vi "Autonomous Independent.vi"() -> ()   [LabVIEW 2018]
doc: "This VI is called when autonomous begins, and will automatically be terminated when autonomous ends. You can carry out timed or sensor driven robot movement independently without needing to return to the caller."
uses:
  <vilib>/Rock Robotics/SystemInterfaces/spilib/spi_bus.ctl
  <vilib>/Rock Robotics/WPI/Utilities/WPI_GetSetVariantRefNum.vi
  <vilib>/Rock Robotics/Network Tables/NT Read String.vi
  <vilib>/Rock Robotics/Network Tables/NT Write Numeric Array.vi
  <vilib>/Rock Robotics/WPI/RobotDrive/WPI_RobotDriveArcadeDrive_Standard(NoSaturation).vi
  <vilib>/Rock Robotics/WPI/Gyro/WPI_GyroXRS450_SPI_Open.vi
panel:
  out "Degrees 2":dbl(knob) scale=0.0..360.0
  in  "Angle 2":dbl=1000.0 min=50.0 max=20000.0 format="%#_13g"
  in  "Angle 1":dbl=1000.0 min=50.0 max=20000.0 format="%#_13g"
  out "Device Found":bool
  in  "SPI Bus":T1
  in  "Sample Rate (Hz)":dbl=1000.0 min=50.0 max=20000.0 format="%#_13g"
  out "Degrees":dbl(knob) scale=0.0..360.0
  in  "Reset Angle?":bool
  out "Calibrated?":bool
  # "This shows wiring for the Analog Devices XRS450 gyro.  It can be plugged directly into the SPI port."
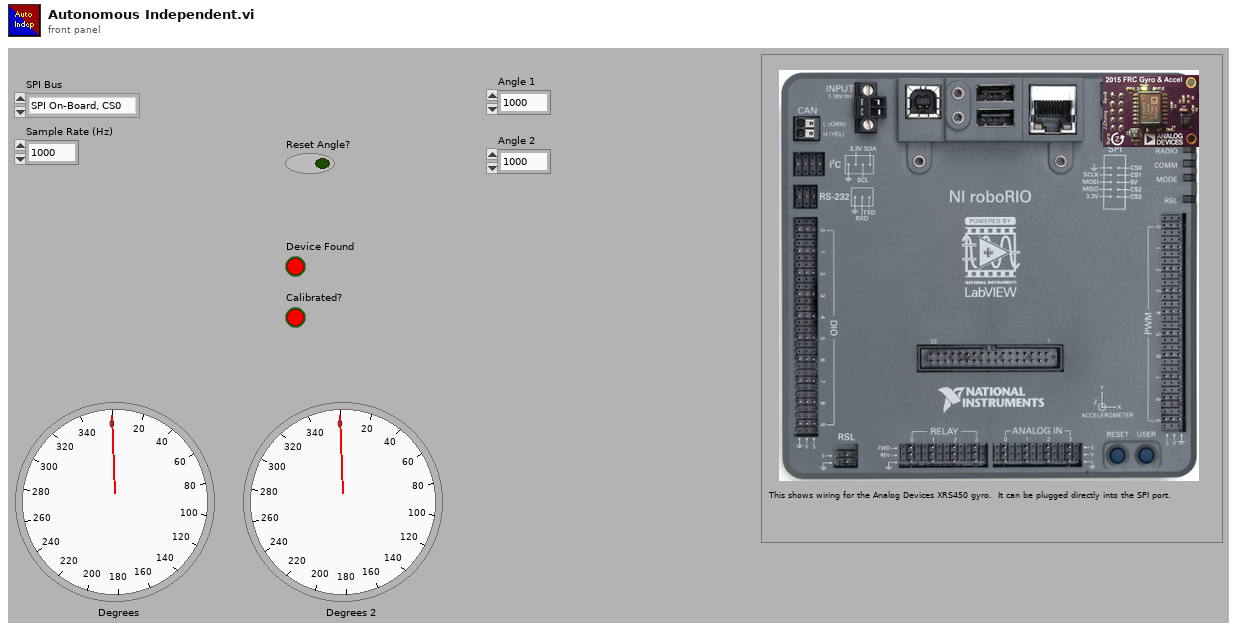
[diagram p1: front panel]
types:
  T1 = typedef "spi_bus.ctl" = enum16{"SPI On-Board, CS0", "SPI On-Board, CS1", "SPI On-Board, CS2", "SPI On-Board, CS3", "SPI MXP", "Invalid"}
  T2 = typedef "WPI_JoystickDevRef.ctl" = cluster{"Device":T3}
  T3 = typedef "WPI_JoystickDeviceEnum.ctl" = enum16{"USB 0", "USB 1", "USB 2", "USB 3", "USB 4", "USB 5"}
  T4 = typedef "WPI_RobotDriveDevRef.ctl" = cluster{"DevStatus":errorcluster, "Motors[]":T5[], "Square Inputs":bool, "Max Output":dbl}
  T5 = typedef "WPI_MotorControlDeviceRef.ctl" = cluster{"DeviceStatus":errorcluster, "Type":T6, "PWM":cluster{"PWM Channel":T7, "DeadBand":T8}, "CAN":cluster{"Device Number":u8, "SetOutput VI Ref":variant, "GetOutput VI Ref":variant, "Enable VI Ref":variant, "Disable VI Ref":variant, "Data":variant}, "Invert":bool, "DIO PWM":cluster{"PWM \"Enable\" Channel":T7, "DIOChannel":T9, "PWM Rate":dbl}}
  T6 = typedef "WPI_MotorControlType.ctl" = enum16{"PWM", "CAN", "DIO PWM"}
  T7 = typedef "FPGA_DIOPWMChannel.ctl" = enum8{"PWM 0", "PWM 1", "PWM 2", "PWM 3", "PWM 4", "PWM 5", "PWM 6", "PWM 7", "PWM 8", "PWM 9", "PWM MXP 0", "PWM MXP 1", "PWM MXP 2", "PWM MXP 3", "PWM MXP 4", "PWM MXP 5", "PWM MXP 6", "PWM MXP 7", "PWM MXP 8", "PWM MXP 9", "Invalid"}
  T8 = typedef "WPI_PWMDeadband.ctl" = cluster{"Name":string, "maxPositivePwm":i32, "minPositivePwm":i32, "centerPwm":i32, "maxNegativePwm":i32, "minNegativePwm":i32, "angularRange":u16}
  T9 = typedef "FPGA_DIOChannel.ctl" = enum8{"DIO 0", "DIO 1", "DIO 2", "DIO 3", "DIO 4", "DIO 5", "DIO 6", "DIO 7", "DIO 8", "DIO 9", "DIO MXP 0", "DIO MXP 1", "DIO MXP 2", "DIO MXP 3", "DIO MXP 4", "DIO MXP 5", "DIO MXP 6", "DIO MXP 7", "DIO MXP 8", "DIO MXP 9", "DIO MXP 10", "DIO MXP 11", "DIO MXP 12", "DIO MXP 13", "DIO MXP 14", "DIO MXP 15", "SPI Port CS1", "SPI Port CS2", "SPI Port CS3", "SPI Port MISO", "SPI Port MOSI", "Invalid"}
  T10 = typedef "WPI_GyroDevRef.ctl" = cluster{"DevStatus":errorcluster, "Analog Channel":T11, "Gain (VoltsPerDegree/Second)":dbl, "Gyro Type":enum16{"Analog", "XRS450"}, "Handle":i32, "SPI Bus":T1, "Device Found":bool, "Sample Rate":dbl, "Calibrate On Open":bool, "Offset":dbl}
  T11 = typedef "FPGA_AIChannel.ctl" = enum8{"AI 0", "AI 1", "AI 2", "AI 3", "AI MXP 0", "AI MXP 1", "AI MXP 2", "AI MXP 3", "Invalid"}
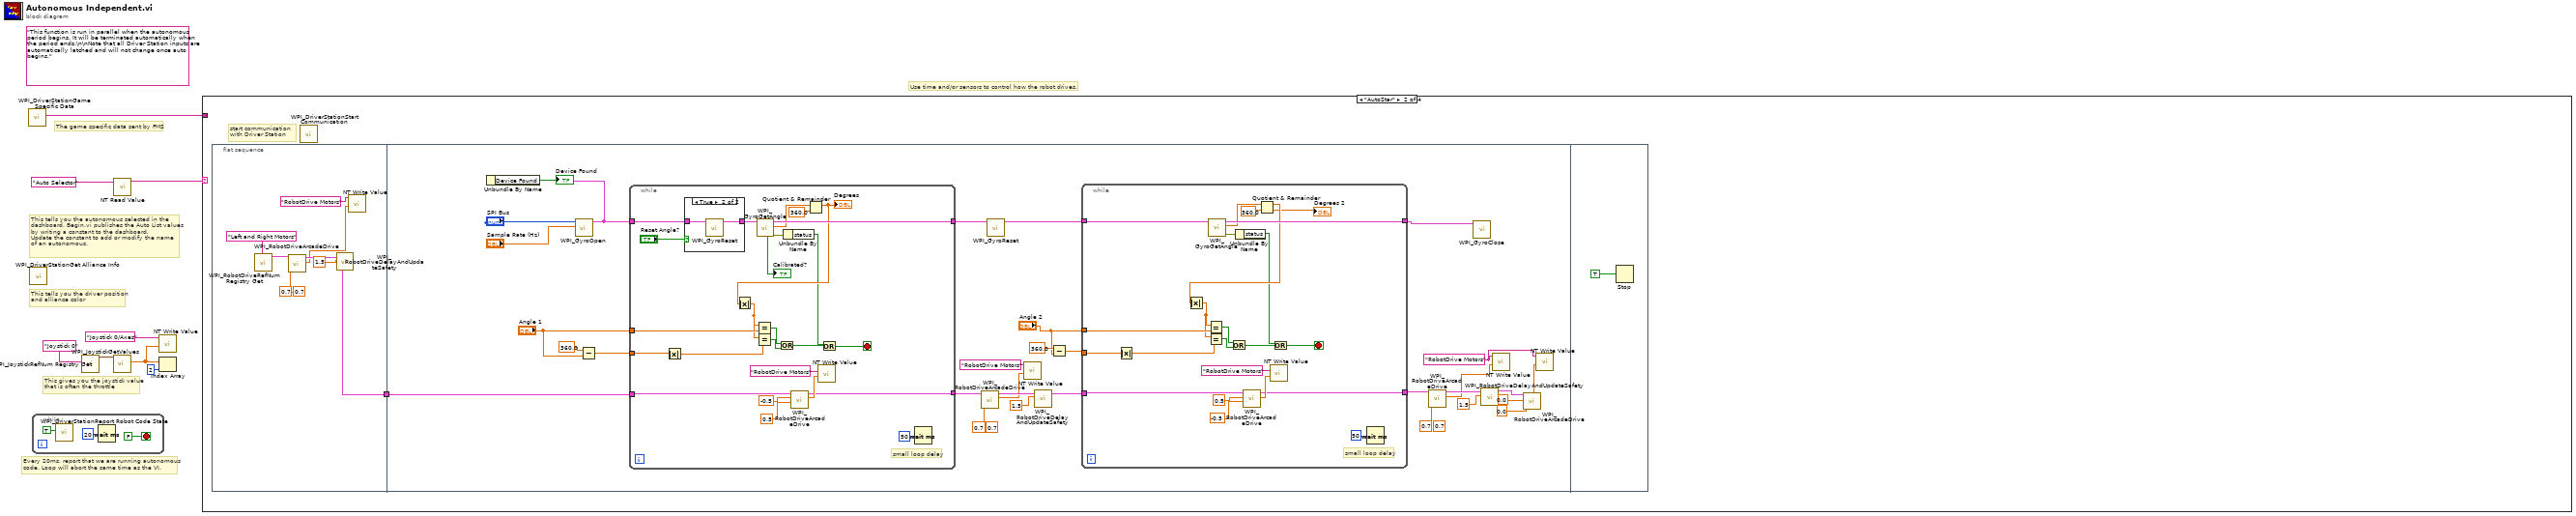
[diagram p0: block diagram]
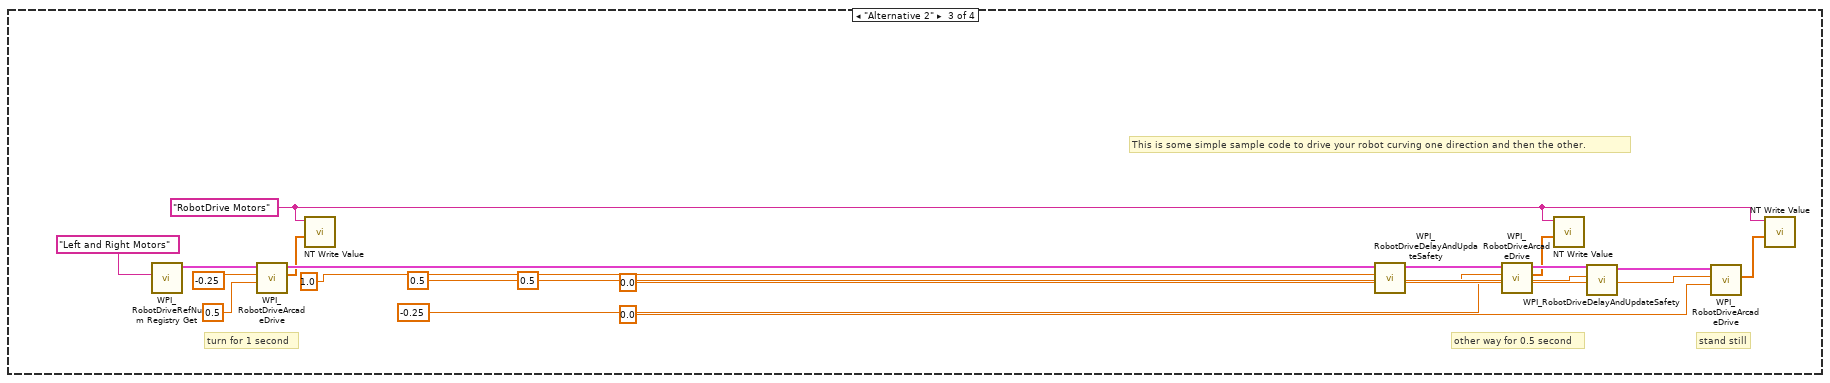
[diagram p4: hidden frame]
diagram:
  (unwired) "This function is run in parallel when the autonomous period begins. It will be terminated automatically when the period ends.\n\nNote that all Driver Station inputs are automatically latched and will not change once auto begins."
  # "The game specific data sent by FMS"
  # "This tells you the autonomous selected in the \ndashboard. Begin.vi publishes the Auto List values\nby writing a constant to the dashboard.\nUpdate the constant to add or modify the name\nof an autonomous."
  # "Every 20ms, report that we are running autonomous\ncode. Loop will abort the same time as the VI."
  # "This gives you the joystick value\nthat is often the throttle"
  # "Use time and/or sensors to control how the robot drives."
  # "This tells you the driver position\nand alliance color"
  n1 = call <vilib>:"WPI_DriverStationGame Specific Data.vi"() -> ("Game Specific Data"=w1:string)  [unwired: 11 in]
  n2 = call <vilib>:"WPI_DriverStationGet Alliance Info.vi"() -> ()  [unwired: 12 out]
  n3 = while {
    stop <- FALSE stop-if-true
    n4 = call <vilib>:"WPI_DriverStationReport Robot Code State.vi"("Autonomous"=TRUE) -> ()  [unwired: 10 in, 1 out]
    n5 = Wait (ms)(milliseconds to wait=u32 20) -> ()  [unwired: 1 out]
  }
  n6 = call <vilib>:"WPI_JoystickRefNum Registry Get.vi"("refnum name"="Joystick 0") -> ("JoystickDevRef"=w7:T2)  [unwired: 1 in, 9 out]
  n7 = call <vilib>:"WPI_JoystickGetValues.vi"("JoystickDevRef"=w7) -> ("Axes"=w3:dbl[])  [unwired: 6 in, 4 out]
  n8 = call-poly <vilib>:"NT Read Value.vi"("Name"="Auto Selector") -> ("String"=w4:string)  [unwired: 9 in, 1 out]
  n9 = call-poly <vilib>:"NT Write Value.vi"("Numeric Array"=w3, "Name"="Joystick 0/Axes") -> ()  [unwired: 9 in, 1 out]
  n10 = Index Array(array=w3, index=2) -> ()  [unwired: 1 out]
  n11 = case shown="\"AutoStar\"" w4 {
    tunnel: w1 -> [_ _ _ _]
    frame Default {
      # "You can put your main auto here, or you can right-click on the case and make any\nother frame be the default case."
      # "This is the frame that will execute if no selection is made, or if it is not recognized"
    }
    frame "AutoStar" {
      # "start communication with Driver Station"
      n12 = flat-sequence {
        tunnel: [w20] -> w12
        tunnel: w12 -> [w50]
        frame #0 {
          n13 = call <vilib>:"WPI_RobotDriveRefNum Registry Get.vi"("refnum name"="Left and Right Motors") -> ("RobotDriveDevRef"=w18:T4)  [unwired: 1 in, 9 out]
          n14 = call-poly <vilib>:"WPI_RobotDriveArcadeDrive.vi"("Y axis value"=0.7, "X axis value"=0.7, "RobotDriveDevRef"=w18) -> ("Motor Values"=w14:dbl[], "RobotDriveDevRef"=w17:T4)  [unwired: 1 in, 6 out]
          n15 = call <vilib>:"WPI_RobotDriveDelayAndUpdateSafety.vi"("Delay (s)"=1.5, "RobotDriveDevRef"=w17) -> ("RobotDriveDevRef 2"=w20:T4)  [unwired: 8 in, 1 out]
          n16 = call-poly <vilib>:"NT Write Value.vi"("Numeric Array"=w14, "Name"="RobotDrive Motors") -> ()  [unwired: 9 in, 1 out]
        }
        frame #1 {
          w26 = "RobotDrive Motors" ("Name")
          n17 = call-poly <vilib>:"WPI_GyroOpen.vi"("Sample Rate (Hz)"="Sample Rate (Hz)", "SPI Bus"="SPI Bus") -> ("GyroDevRef"=w53:T10)  [unwired: 7 in, 2 out]
          n18 = Unbundle By Name(w53) -> ("Device Found"=→"Device Found":bool)
          n19 = Subtract(x=360.0, y="Angle 1") -> (x-y=w47:dbl)
          n20 = while {
            tunnel: w53 -> [w99]
            tunnel: [w97] -> w41
            tunnel: "Angle 1" -> [w82]
            tunnel: w50 -> [w88]
            tunnel: w47 -> [w83]
            tunnel: [w80] -> w42
            stop <- w93 stop-if-true
            # "small loop delay"
            n21 = Absolute Value(x=w83) -> (abs(x)=w79:dbl)
            n22 = case shown="True" "Reset Angle?" {
              tunnel: w99 -> [w103 w105]
              tunnel: [w103 w104] -> w98
              frame False {
              }
              frame True {
                n23 = call <vilib>:"WPI_GyroReset.vi"("GyroDevRef"=w105) -> ("GyroDevRef"=w104:T10)  [unwired: 9 in, 1 out]
              }
            }
            n24 = call <vilib>:"WPI_GyroGetAngle.vi"("GyroDevRef"=w98) -> ("error out"=w95:errorcluster, "Angle"=w96:dbl, "GyroDevRef"=w97:T10, "Calibrated?"=→"Calibrated?":bool)  [unwired: 6 in, 1 out]
            n25 = Unbundle By Name(w95) -> ("status"=w78:bool)
            n26 = call-poly <vilib>:"WPI_RobotDriveArcadeDrive.vi"("Y axis value"=0.5 ("X axis value"), "X axis value"=-0.5, "RobotDriveDevRef"=w88) -> ("Motor Values"=w92:dbl[], "RobotDriveDevRef"=w80:T4)  [unwired: 1 in, 6 out]
            n27 = Quotient & Remainder(x=w96, y=360.0) -> (x-y*floor(x/y)=w87:dbl)  [unwired: 1 out]
            "Degrees" <- w87
            n28 = Absolute Value(x=w87) -> (abs(x)=w81:dbl)
            n29 = Equal?(x=w81, y=w82) -> (x = y?=w86:bool)
            n30 = Equal?(x=w81, y=w79) -> (x = y?=w84:bool)
            n31 = Or(x=w86, y=w84) -> (x .or. y?=w85:bool)
            n32 = call-poly <vilib>:"NT Write Value.vi"("Numeric Array"=w92, "Name"="RobotDrive Motors") -> ()  [unwired: 9 in, 1 out]
            n33 = Or(x=w78, y=w85) -> (x .or. y?=w93:bool)
            n34 = Wait (ms)(milliseconds to wait=u32 50) -> ()  [unwired: 1 out]
          }
          n35 = call-poly <vilib>:"WPI_RobotDriveArcadeDrive.vi"("Y axis value"=0.7, "X axis value"=0.7, "RobotDriveDevRef"=w42) -> ("Motor Values"=w29:dbl[], "RobotDriveDevRef"=w45:T4)  [unwired: 1 in, 6 out]
          n36 = call <vilib>:"WPI_GyroReset.vi"("GyroDevRef"=w41) -> ("GyroDevRef"=w40:T10)  [unwired: 9 in, 1 out]
          n37 = call-poly <vilib>:"NT Write Value.vi"("Numeric Array"=w29, "Name"="RobotDrive Motors") -> ()  [unwired: 9 in, 1 out]
          n38 = call <vilib>:"WPI_RobotDriveDelayAndUpdateSafety.vi"("Delay (s)"=1.5, "RobotDriveDevRef"=w45) -> ("RobotDriveDevRef 2"=w39:T4)  [unwired: 8 in, 1 out]
          n39 = Subtract(x=360.0, y="Angle 2") -> (x-y=w38:dbl)
          n40 = while {
            tunnel: w40 -> [w55]
            tunnel: [w75] -> w22
            tunnel: "Angle 2" -> [w61]
            tunnel: w39 -> [w67]
            tunnel: w38 -> [w62]
            tunnel: [w59] -> w31
            stop <- w72 stop-if-true
            # "small loop delay"
            n41 = Absolute Value(x=w62) -> (abs(x)=w58:dbl)
            n42 = call <vilib>:"WPI_GyroGetAngle.vi"("GyroDevRef"=w55) -> ("error out"=w73:errorcluster, "Angle"=w74:dbl, "GyroDevRef"=w75:T10)  [unwired: 6 in, 2 out]
            n43 = Unbundle By Name(w73) -> ("status"=w57:bool)
            n44 = call-poly <vilib>:"WPI_RobotDriveArcadeDrive.vi"("Y axis value"=-0.5 ("X axis value"), "X axis value"=0.5, "RobotDriveDevRef"=w67) -> ("Motor Values"=w71:dbl[], "RobotDriveDevRef"=w59:T4)  [unwired: 1 in, 6 out]
            n45 = Quotient & Remainder(x=w74, y=360.0) -> (x-y*floor(x/y)=w66:dbl, floor(x/y)=→"Degrees 2":dbl)
            n46 = Absolute Value(x=w66) -> (abs(x)=w60:dbl)
            n47 = Equal?(x=w60, y=w61) -> (x = y?=w65:bool)
            n48 = Equal?(x=w60, y=w58) -> (x = y?=w63:bool)
            n49 = Or(x=w65, y=w63) -> (x .or. y?=w64:bool)
            n50 = call-poly <vilib>:"NT Write Value.vi"("Numeric Array"=w71, "Name"="RobotDrive Motors") -> ()  [unwired: 9 in, 1 out]
            n51 = Or(x=w57, y=w64) -> (x .or. y?=w72:bool)
            n52 = Wait (ms)(milliseconds to wait=u32 50) -> ()  [unwired: 1 out]
          }
          n53 = call-poly <vilib>:"WPI_RobotDriveArcadeDrive.vi"("Y axis value"=0.7, "X axis value"=0.7, "RobotDriveDevRef"=w31) -> ("Motor Values"=w27:dbl[], "RobotDriveDevRef"=w34:T4)  [unwired: 1 in, 6 out]
          n54 = call <vilib>:"WPI_GyroClose.vi"("GyroDevRef"=w22) -> ()  [unwired: 10 in, 1 out]
          n55 = call <vilib>:"WPI_RobotDriveDelayAndUpdateSafety.vi"("Delay (s)"=1.5, "RobotDriveDevRef"=w34) -> ("RobotDriveDevRef 2"=w30:T4)  [unwired: 8 in, 1 out]
          n56 = call-poly <vilib>:"NT Write Value.vi"("Numeric Array"=w27, "Name"=w26) -> ()  [unwired: 9 in, 1 out]
          n57 = call-poly <vilib>:"WPI_RobotDriveArcadeDrive.vi"("Y axis value"=0.0, "X axis value"=0.0, "RobotDriveDevRef"=w30) -> ("Motor Values"=w25:dbl[])  [unwired: 1 in, 7 out]
          n58 = call-poly <vilib>:"NT Write Value.vi"("Numeric Array"=w25, "Name"=w26) -> ()  [unwired: 9 in, 1 out]
        }
        frame #2 {
          n59 = Stop(stop? (T)=TRUE) -> ()
        }
      }
      n60 = call <vilib>:"WPI_DriverStationStart Communication.vi"() -> ()  [unwired: 12 in]
    }
    frame "Alternative 2" {
      w108 = "RobotDrive Motors" ("Name")
      # "This is some simple sample code to drive your robot curving one direction and then the other."
      # "stand still"
      # "other way for 0.5 second"
      # "turn for 1 second"
      n61 = call <vilib>:"WPI_RobotDriveRefNum Registry Get.vi"("refnum name"="Left and Right Motors") -> ("RobotDriveDevRef"=w124:T4)  [unwired: 1 in, 9 out]
      n62 = call-poly <vilib>:"WPI_RobotDriveArcadeDrive.vi"("Y axis value"=0.5 ("X axis value"), "X axis value"=-0.25, "RobotDriveDevRef"=w124) -> ("Motor Values"=w107:dbl[], "RobotDriveDevRef"=w117:T4)  [unwired: 1 in, 6 out]
      n63 = call-poly <vilib>:"NT Write Value.vi"("Numeric Array"=w107, "Name"=w108) -> ()  [unwired: 9 in, 1 out]
      n64 = call <vilib>:"WPI_RobotDriveDelayAndUpdateSafety.vi"("Delay (s)"=1.0, "RobotDriveDevRef"=w117) -> ("RobotDriveDevRef 2"=w118:T4)  [unwired: 8 in, 1 out]
      n65 = call-poly <vilib>:"WPI_RobotDriveArcadeDrive.vi"("Y axis value"=-0.25 ("X axis value"), "X axis value"=0.5, "RobotDriveDevRef"=w118) -> ("Motor Values"=w109:dbl[], "RobotDriveDevRef"=w119:T4)  [unwired: 1 in, 6 out]
      n66 = call-poly <vilib>:"NT Write Value.vi"("Numeric Array"=w109, "Name"=w108) -> ()  [unwired: 9 in, 1 out]
      n67 = call <vilib>:"WPI_RobotDriveDelayAndUpdateSafety.vi"("Delay (s)"=0.5, "RobotDriveDevRef"=w119) -> ("RobotDriveDevRef 2"=w120:T4)  [unwired: 8 in, 1 out]
      n68 = call-poly <vilib>:"WPI_RobotDriveArcadeDrive.vi"("Y axis value"=0.0 ("X axis value"), "X axis value"=0.0, "RobotDriveDevRef"=w120) -> ("Motor Values"=w110:dbl[])  [unwired: 1 in, 7 out]
      n69 = call-poly <vilib>:"NT Write Value.vi"("Numeric Array"=w110, "Name"=w108) -> ()  [unwired: 9 in, 1 out]
    }
    frame "Your Turn" {
    }
  }
